vi "HB_ReadDIOAllChannels.vi"(8 "error in (no error)":errorcluster, 11 "HBDeviceRef":T1) -> (0 "error out":errorcluster, 2 "All Digital Input Vals":bool[](array[boolean]), 3 "HBDeviceRef":T1)   [LabVIEW 2018]
doc: "Reads all 32 DIO channels on the Huskie Board and returns the current values."
uses:
  <vilib>/Rock Robotics/WPI/SerialPort/WPI_SerialPortRef.ctl
  <vilib>/Utility/error.llb/Error Cluster From Error Code.vi
  <vilib>/ErrorRing/Error Ring.xnode
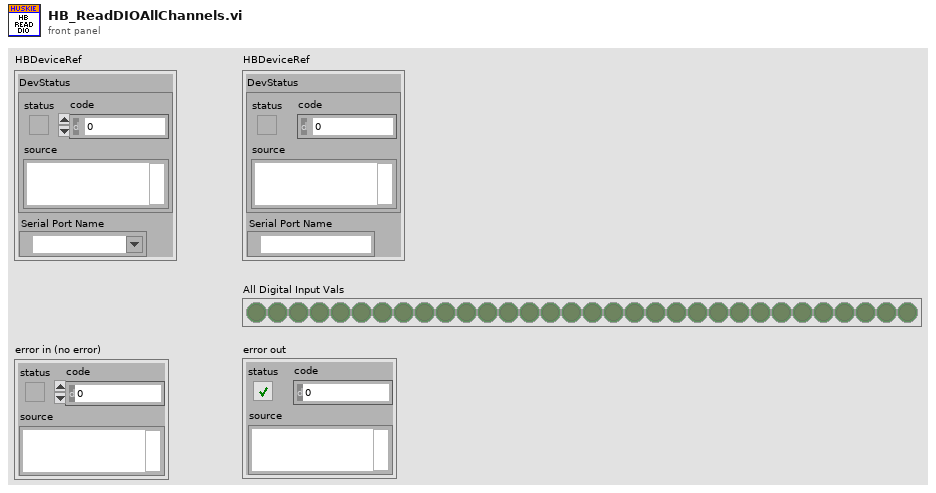
[diagram p1: front panel]
types:
  T1 = typedef "WPI_SerialPortRef.ctl" = cluster{"DevStatus":errorcluster, "Serial Port Name":refnum<visa-resource-name>}
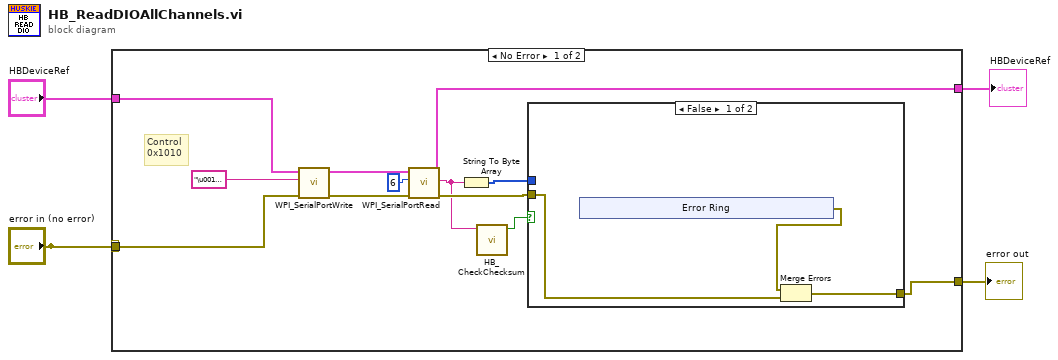
[diagram p0: block diagram]
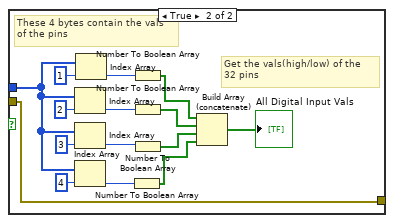
[diagram p2: hidden frame]
diagram:
  n1 = case shown="No Error" "error in (no error)" {
    selector: "error in (no error)" -> [_ w39]
    tunnel: "HBDeviceRef" -> [w16 w40]
    tunnel: [w15 w40] -> w3
    tunnel: "error in (no error)" -> [w14 _]
    tunnel: [w8 w39] -> w2
    frame No Error {
      # "Control\n0x1010"
      n2 = call <vilib>:"WPI_SerialPortWrite.vi"("error in (no error)"=w14, "Buffer"="\u0010\u0010", "SerialPortRef"=w16) -> ("error out"=w12:errorcluster, "SerialPortRef"=w13:T1)  [unwired: 6 in, 1 out]
      n3 = call <vilib>:"WPI_SerialPortRead.vi"("error in (no error)"=w12, "Num Bytes to Read"=u32 6, "SerialPortRef"=w13) -> ("error out"=w9:errorcluster, "Buffer"=w6:string, "SerialPortRef"=w15:T1)  [unwired: 6 in]
      n4 = String To Byte Array(string=w6) -> (unsigned byte array=w7:u8[])
      n5 = call <vilib>:"HB_CheckChecksum.vi"("String"=w6) -> ("Checksum Matches"=w5:bool)  [unwired: 9 in, 1 out]
      n6 = case shown="False" w5 {
        tunnel: w7 -> [_ w25]
        tunnel: w9 -> [w19 w24]
        tunnel: [w18 w24] -> w8
        frame False {
          n7 = xnode "Error Ring"() -> ("error out"=w17:errorcluster)
          n8 = Merge Errors(w17, w19) -> (w18:errorcluster)
        }
        frame True {
          # "These 4 bytes contain the vals \nof the pins"
          # "Get the vals(high/low) of the \n32 pins"
          n9 = Index Array(array=w25, index=2) -> (element=w31:u8)
          n10 = Index Array(array=w25, index=3) -> (element=w32:u8)
          n11 = Index Array(array=w25, index=4) -> (element=w33:u8)
          n12 = Index Array(array=w25, index=1) -> (element=w34:u8)
          n13 = Number To Boolean Array(number=w33) -> (Boolean array=w27:bool[])
          n14 = Number To Boolean Array(number=w34) -> (Boolean array=w30:bool[])
          n15 = Number To Boolean Array(number=w31) -> (Boolean array=w29:bool[])
          n16 = Number To Boolean Array(number=w32) -> (Boolean array=w28:bool[])
          n17 = Build Array (concatenate)(w30, w29, w28, w27) -> (→"All Digital Input Vals":bool[])
        }
      }
    }
    frame Error {
    }
  }
  "HBDeviceRef" <- w3
  "error out" <- w2
